vi "Normalize Name.vi"(10 "Action Name":string) -> (2 "Normalized Name":string)   [LabVIEW 2020, in "neg-pkg.lvlib" / "Action.lvclass"]
uses:
  Action.lvclass
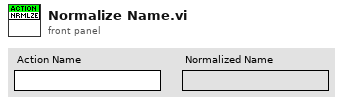
[diagram p1: front panel]
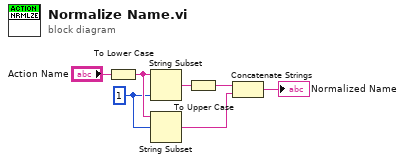
[diagram p0: block diagram]
diagram:
  w5 = 1 ("length (rest)")
  n1 = To Lower Case(string="Action Name") -> (all lower case string=w6:string)
  n2 = String Subset(string=w6, length (rest)=w5) -> (substring=w4:string)  [unwired: 1 in]
  n3 = String Subset(string=w6, offset (0)=w5) -> (substring=w2:string)  [unwired: 1 in]
  n4 = To Upper Case(1:w4) -> (0:w3:string)
  n5 = Concatenate Strings(w3, w2) -> (→"Normalized Name":string)
